vi "Item Info To Tree.vi"(7 "Owning Tree":string, 8 "error in":errorcluster, 9 "Config File":path, 10 "Item Info":T2[](array[typedef]), 11 "Tree Manager in":T1) -> (0 "error out":errorcluster, 3 "Tree Manager out":T1)   [LabVIEW 2020]
uses:
  <vilib>/addons/analyzer/_vianuishared.llb/VIAnUI Item Info.ctl
  <vilib>/addons/analyzer/_vianuishared.llb/VIAnUI Path Type.ctl
  <vilib>/addons/analyzer/VIAnCFGDataStructure/Tree Manager/Typedefs/Session Handle.ctl
  <vilib>/addons/analyzer/VIAnCFGDataStructure/Tree Manager/Tree.lvclass
  <vilib>/addons/analyzer/VIAnCFGDataStructure/Data Types/Bool/Bool.lvclass/Bool.ctl
  <vilib>/addons/analyzer/VIAnCFGDataStructure/Data Types/Path/Path.lvclass/Path.ctl
  <vilib>/addons/analyzer/VIAnCFGDataStructure/Data Types/Path/To Path Tree Data.vi
  <vilib>/addons/analyzer/VIAnCFGDataStructure/Data Types/Bool/To Bool Tree Data.vi
  <vilib>/addons/analyzer/VIAnCFGDataStructure/Data Types/Path/Path.lvclass
  e:/builds/penguin/labview/branches/2020/dev/dist/vi.lib/addons/analyzer/VIAnCFGDataStructure/Tree Data/Tree Data.lvclass
  <vilib>/addons/analyzer/VIAnCFGDataStructure/Data Types/Bool/Bool.lvclass
  <vilib>/addons/analyzer/_vianuishared.llb/VIAnUI CFG File Info Global.vi
  <vilib>/addons/analyzer/VIAnCFGDataStructure/Tree Manager/API/Set Attribute Tree Data.vi
  e:/builds/penguin/labview/branches/2020/dev/dist/vi.lib/addons/analyzer/VIAnCFGDataStructure/Data Types/Path/Path.lvclass
  e:/builds/penguin/labview/branches/2020/dev/dist/vi.lib/addons/analyzer/VIAnCFGDataStructure/Data Types/Bool/Bool.lvclass
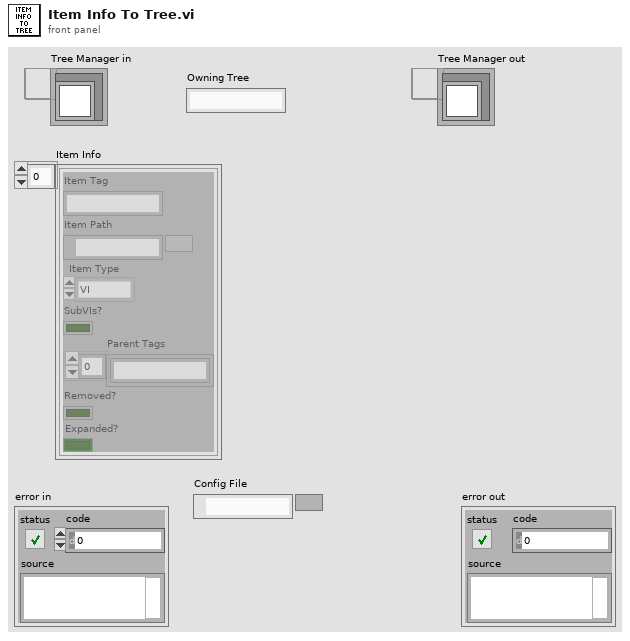
[diagram p1: front panel]
types:
  T1 = typedef "NI_VIAnCFGDataStructure.lvlib/Tree.lvclass/Session Handle.ctl" = refnum<data-value>
  T2 = typedef "VIAnUI Item Info.ctl" = cluster{"Item Tag":string, "Item Path":path, "Item Type":T3, "SubVIs?":bool, "Parent Tags":string[], "Removed?":bool, "Expanded?":bool}
  T3 = typedef "VIAnUI Path Type.ctl" = enum16{"VI", "LLB", "Folder", "Invalid", "ProjItem"}
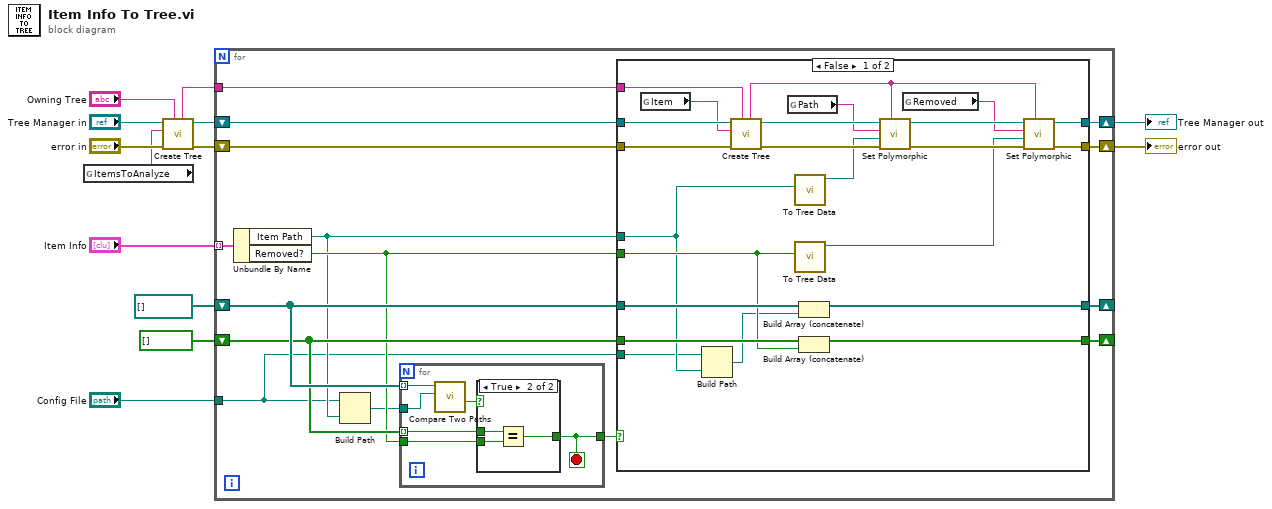
[diagram p0: block diagram]
diagram:
  n1 = global read "VIAnUI CFG File Info Global.vi" "ItemsToAnalyze"() -> (w5:string)
  n2 = call <vilib>:"Create Tree.vi"("Parent ID (empty)"="Owning Tree", "Error In"="error in", "Name"=w5, "Tree Manager"="Tree Manager in") -> ("Error Out"=w9:errorcluster, "Tree Manager"=w10:T1, "Unique ID"=w8:string)  [unwired: 5 in]
  n3 = for {
    tunnel: "Item Info" -> [w28] mode=indexing
    shift-right: [w24] -> w6
    shift-left: w10 -> [w27]
    shift-right: [w23] -> w13
    shift-left: w9 -> [w26]
    tunnel: w8 -> [w25]
    shift-right: [w21] -> _
    shift-left: path[] [] -> [w22]
    shift-right: [w20] -> _
    shift-left: bool[] [] -> [w19]
    tunnel: "Config File" -> [w14]
    n4 = Unbundle By Name(w28) -> ("Item Path"=w16:path, "Removed?"=w18:bool)
    n5 = Build Path(base path=w14, name or relative path=w16) -> (appended path=w15:path)
    n6 = for {
      tunnel: w22 -> [w34] mode=indexing
      tunnel: w15 -> [w33]
      tunnel: w19 -> [w31] mode=indexing
      tunnel: w18 -> [w30]
      tunnel: [w29] -> w17
      stop <- w29 stop-if-true
      n7 = call <vilib>:"Compare Two Paths.vi"("Path 2"=w33, "Path 1"=w34) -> ("Path 2 Relative to Path 1?"=w32:bool)  [unwired: 6 in, 3 out]
      n8 = case shown="True" w32 {
        selector: w32 -> [w35 _]
        tunnel: w31 -> [_ w38]
        tunnel: w30 -> [_ w37]
        tunnel: [w35 w36] -> w29
        frame False {
        }
        frame True {
          n9 = Equal?(x=w38, y=w37) -> (x = y?=w36:bool)
        }
      }
    }
    n10 = case shown="False" w17 {
      tunnel: w27 -> [w57 w63]
      tunnel: w26 -> [w56 w62]
      tunnel: w25 -> [w55 _]
      tunnel: [w54 w63] -> w24
      tunnel: [w53 w62] -> w23
      tunnel: w18 -> [w42 _]
      tunnel: w16 -> [w40 _]
      tunnel: w22 -> [w46 w65]
      tunnel: w19 -> [w44 w64]
      tunnel: [w45 w65] -> w21
      tunnel: [w43 w64] -> w20
      tunnel: w14 -> [w39 _]
      frame False {
        n11 = global read "VIAnUI CFG File Info Global.vi" "Item"() -> (w49:string)
        n12 = Build Path(base path=w39, name or relative path=w40) -> (appended path=w41:path)
        n13 = call <vilib>:"Create Tree.vi"("Parent ID (empty)"=w55, "Error In"=w56, "Name"=w49, "Tree Manager"=w57) -> ("Error Out"=w60:errorcluster, "Tree Manager"=w61:T1, "Unique ID"=w52:string)  [unwired: 5 in]
        n14 = global read "VIAnUI CFG File Info Global.vi" "Path"() -> (w48:string)
        n15 = call-poly <vilib>:"To Tree Data.vi"("Path"=w40) -> ("Path Tree Data"=w51:refnum<class "Path.lvclass">)  [unwired: 10 in]
        n16 = call-poly <vilib>:"To Tree Data.vi"("Boolean"=w42) -> ("Bool Tree Data"=w50:refnum<class "Bool.lvclass">)  [unwired: 10 in]
        n17 = Build Array (concatenate)(w46, w41) -> (w45:path[])
        n18 = Build Array (concatenate)(w44, w42) -> (w43:bool[])
        n19 = call-poly <vilib>:"Set Polymorphic.vi"("Tree ID"=w52, "Error In"=w60, "Attribute Value"=w51, "Attribute Name"=w48, "Tree Manager"=w61) -> ("Error Out"=w58:errorcluster, "Tree Manager"=w59:T1)  [unwired: 4 in, 1 out]
        n20 = global read "VIAnUI CFG File Info Global.vi" "Removed"() -> (w47:string)
        n21 = call-poly <vilib>:"Set Polymorphic.vi"("Tree ID"=w52, "Error In"=w58, "Attribute Value"=w50, "Attribute Name"=w47, "Tree Manager"=w59) -> ("Error Out"=w53:errorcluster, "Tree Manager"=w54:T1)  [unwired: 4 in, 1 out]
      }
      frame True {
        # "This path already has a parent in the list that shares the same 'Removed' setting. No need to add it to the XML."
      }
    }
  }
  "error out" <- w13
  "Tree Manager out" <- w6
